vi "RT Error Handler - DAQ Control.vi"(8 "error in (no error)":errorcluster, 11 "Message Queue":refnum<queue>) -> (2 "Enqueued Error?":bool, 3 "dup Message Queue":refnum<queue>)   [LabVIEW 2022 SP3]
uses:
  support/Message Queue/Message Cluster.ctl
  controls/Error Type.ctl
  support/Message Queue/Message Queue.lvlib
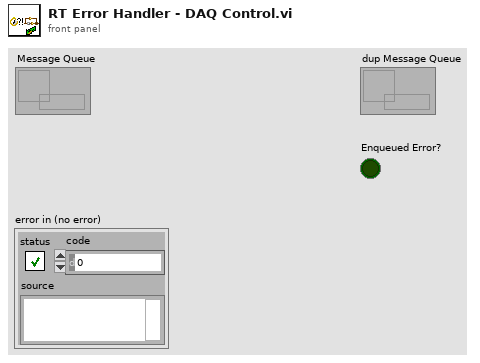
[diagram p1: front panel]
types:
  T1 = typedef "Error Type.ctl" = enum16{"Log-Only Error", "Non-Critical Error", "Critical Error"}
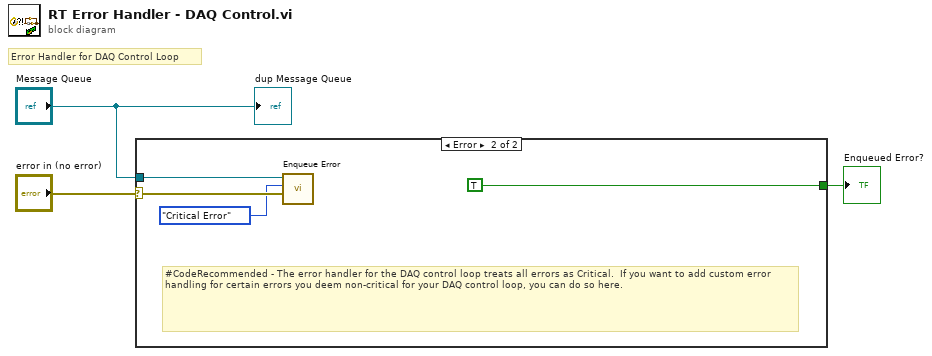
[diagram p0: block diagram]
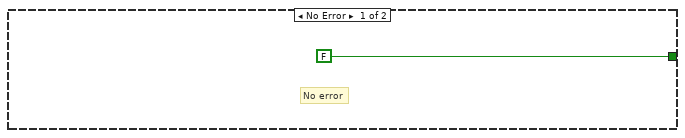
[diagram p2: hidden frame]
diagram:
  # "Error Handler for DAQ Control Loop"
  n1 = case shown="Error" "error in (no error)" {
    selector: "error in (no error)" -> [_ w7]
    tunnel: "Message Queue" -> [_ w8]
    tunnel: [FALSE ("Enqueued Error?") TRUE ("Enqueued Error?")] -> w2
    frame No Error {
      # "No error"
    }
    frame Error {
      # "#CodeRecommended - The error handler for the DAQ control loop treats all errors as Critical.  If you want to add custom error handling for certain errors you deem non-critical for your DAQ control loop, you can do so here."
      n2 = call "Enqueue Error.vi"("error to process"=w7, "Error Type (Non-Critical)"=Error_Type."Critical Error", "Message Queue"=w8) -> ()  [unwired: 9 in]
    }
  }
  "Enqueued Error?" <- w2
  "dup Message Queue" <- "Message Queue"
